vi "cumplimiento_int.vi"(8 "error in (no error)":errorcluster, 11 "Prueba08 in":refnum<class "Prueba031.lvclass">) -> (0 "error out":errorcluster, 2 "cumpimiento":string, 3 "Prueba08 out":refnum<class "Prueba031.lvclass">)   [LabVIEW 2019, in "Prueba031.lvclass"]
uses:
  Prueba031.lvclass
  Prueba031.lvclass/Prueba031.ctl
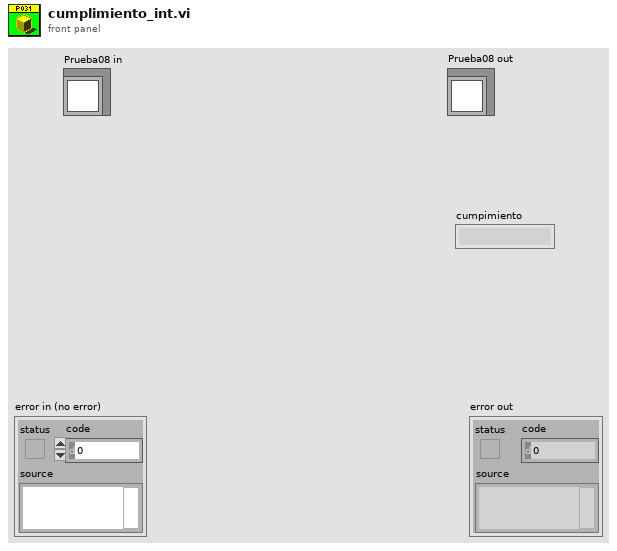
[diagram p1: front panel]
types:
  T1 = cluster{"Medido":dbl, "Medido_Cor":dbl, "Error":dbl, "Ref":dbl, "Incert_exp":dbl, "Tol+":dbl, "Tol-":dbl, "fila":i32}
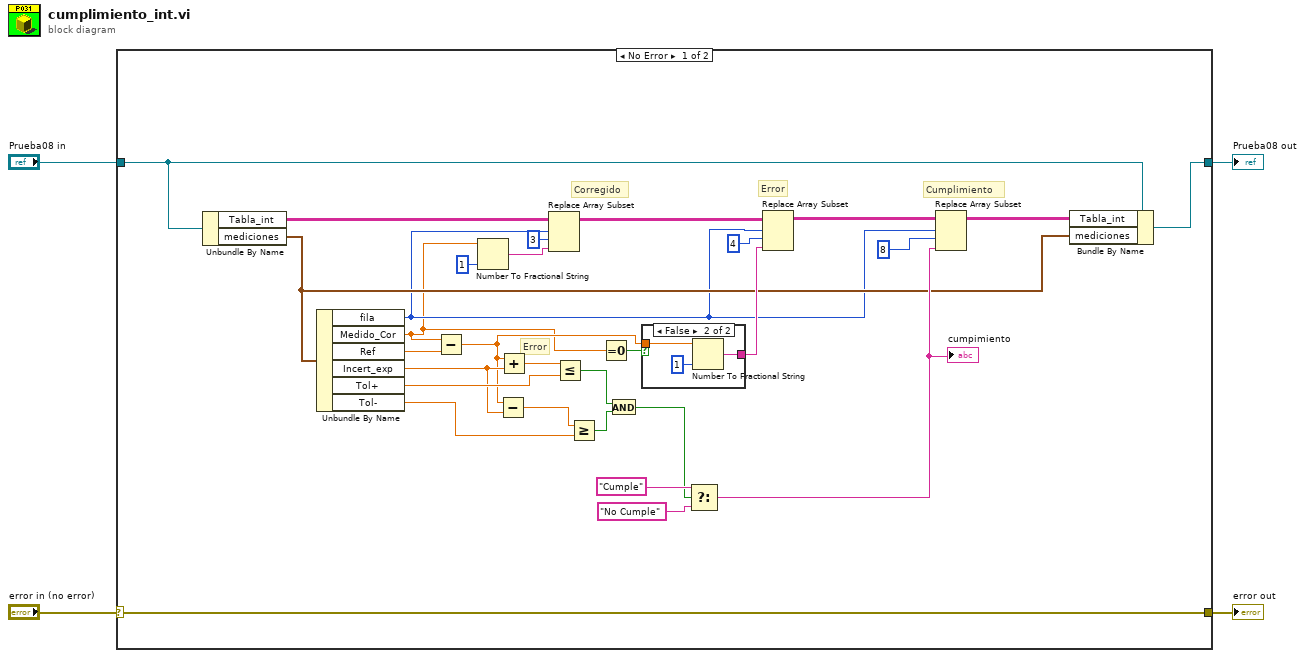
[diagram p0: block diagram]
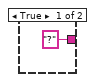
[diagram p2: hidden frame]
diagram:
  n1 = case shown="No Error" "error in (no error)" {
    selector: "error in (no error)" -> [w34 w40]
    tunnel: [w34 w40] -> w3
    tunnel: [w16 w39] -> w2
    tunnel: "Prueba08 in" -> [w13 w39]
    frame No Error {
      # "Corregido"
      # "Cumplimiento"
      # "Error"
      # "Error"
      n2 = Unbundle By Name(w13) -> ("Tabla_int"=w11:string[][], "mediciones"=w14:T1)
      n3 = Unbundle By Name(w14) -> ("fila"=w9:i32, "Medido_Cor"=w5:dbl, "Ref"=w27:dbl, "Incert_exp"=w25:dbl, "Tol+"=w26:dbl, "Tol-"=w24:dbl)
      n4 = Subtract(x=w5, y=w27) -> (x-y=w17:dbl)
      n5 = Number To Fractional String(number=w5, precision (6)=i16 1) -> (F-format string=w6:string)  [unwired: 2 in]
      n6 = Subtract(x=w17, y=w25) -> (x-y=w30:dbl)
      n7 = Add(x=w17, y=w25) -> (x+y=w33:dbl)
      n8 = Replace Array Subset(array=w11, new element=w6, index (row)=w9, index (col)=3 ("disabled index (col)")) -> (w10:string[][])
      n9 = Less Or Equal?(x=w33, y=w26) -> (x <= y?=w32:bool)
      n10 = Greater Or Equal?(x=w30, y=w24) -> (x >= y?=w31:bool)
      n11 = Equal To 0?(x=w5) -> (x = 0?=w18:bool)
      n12 = And(x=w32, y=w31) -> (x .and. y?=w12:bool)
      n13 = case shown="False" w18 {
        tunnel: w17 -> [_ w38]
        tunnel: ["?" w36] -> w19
        frame True {
        }
        frame False {
          n14 = Number To Fractional String(number=w38, precision (6)=i16 1) -> (F-format string=w36:string)  [unwired: 2 in]
        }
      }
      n15 = Select(t="Cumple", s=w12, f="No Cumple") -> (s? t:f=w23:string)
      "cumpimiento" <- w23
      n16 = Replace Array Subset(array=w10, new element=w19, index (row)=w9, index (col)=4 ("disabled index (col)")) -> (w21:string[][])
      n17 = Replace Array Subset(array=w21, new element=w23, index (row)=w9, index (col)=8 ("index (row)")) -> (w15:string[][])
      n18 = Bundle By Name(cluster=w13, "Tabla_int"=w15, "mediciones"=w14) -> (w16:refnum<class "Prueba031.lvclass">)
    }
    frame Error {
    }
  }
  "error out" <- w3
  "Prueba08 out" <- w2
